vi "Valid Number.vi"(3 "Number":dbl) -> (5 "Valid":bool)   [LabVIEW 2021, in "DataTypes_CIF_U.lvlib"]
uses:
  DataTypes_CIF_U.lvlib
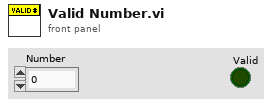
[diagram p1: front panel]
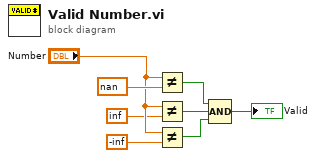
[diagram p0: block diagram]
diagram:
  n1 = Not Equal?(x="Number", y=nan) -> (x != y?=w6:bool)
  n2 = Not Equal?(x="Number", y=inf) -> (x != y?=w1:bool)
  n3 = Not Equal?(x="Number", y=-inf) -> (x != y?=w2:bool)
  n4 = Compound Arithmetic op=AND(w6, w1, w2) -> (→"Valid":bool)
